vi "port_readline.vi"(8 "error in (no error)":errorcluster, 10 "String in":string, 11 "VISA Refnum in":refnum<visa-resource-name>) -> (0 "error out":errorcluster, 2 "reply":string, 3 "VISA Refnum out":refnum<visa-resource-name>)   [LabVIEW 2024]
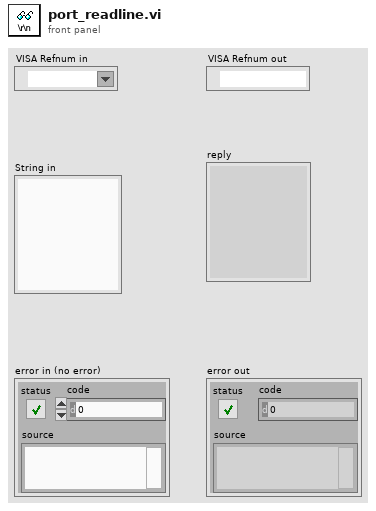
[diagram p1: front panel]
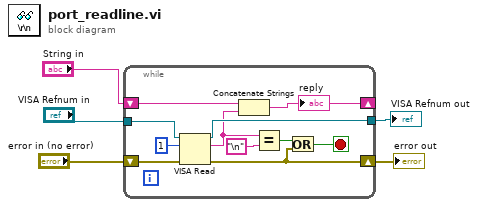
[diagram p0: block diagram]
diagram:
  n1 = while {
    tunnel: "VISA Refnum in" -> [w16]
    tunnel: [w13] -> w3
    shift-right: [w10] -> w5
    shift-left: "error in (no error)" -> [w12]
    shift-right: [w6] -> _
    shift-left: "String in" -> [w7]
    stop <- w9 stop-if-true
    n2 = VISA Read(VISA resource name=w16, byte count=u32 1, error in (no error)=w12) -> (VISA resource name out=w13:refnum<visa-resource-name>, read buffer=w8:string, error out=w10:errorcluster)  [unwired: 1 out]
    n3 = Concatenate Strings(w7, w8) -> (w6:string)
    "reply" <- w6
    n4 = Equal?(x=w8, y="\n") -> (x = y?=w11:bool)
    n5 = Or(x=w11, y=w10) -> (x .or. y?=w9:bool)
  }
  "error out" <- w5
  "VISA Refnum out" <- w3
